vi "CreateNotifiers.vi"(8 "error in":errorcluster) -> (0 "error out":errorcluster, 3 "Notifiers":T1)   [LabVIEW 2015]
uses:
  Notifiers.ctl
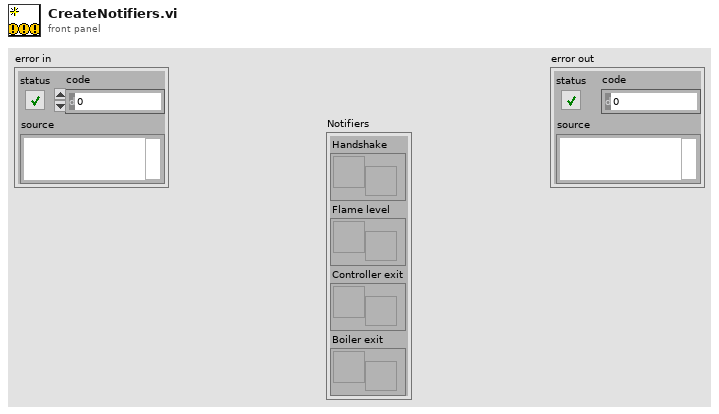
[diagram p1: front panel]
types:
  T1 = typedef "Notifiers.ctl" = cluster{"Handshake":refnum<notifier>, "Flame level":refnum<notifier>, "Controller exit":refnum<notifier>, "Boiler exit":refnum<notifier>}
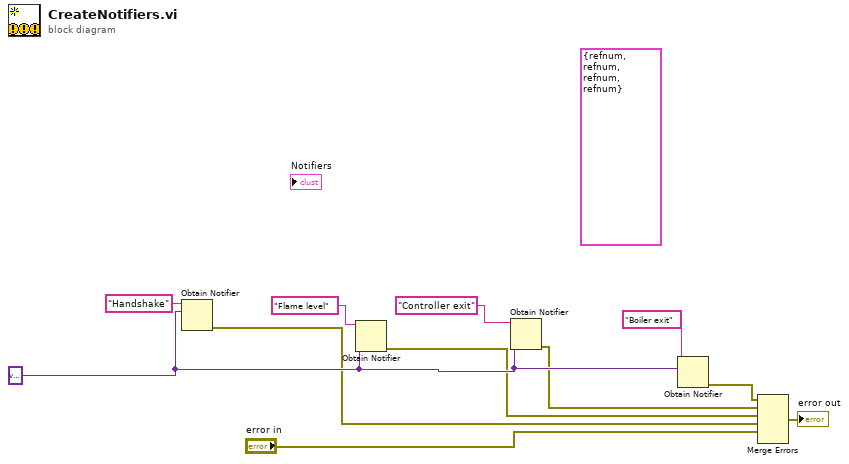
[diagram p0: block diagram]
diagram:
  (unwired) T1 {"Handshake"=refnum, "Flame level"=refnum, "Controller exit"=refnum, "Boiler exit"=refnum}
  w7 = variant
  n1 = Obtain Notifier(name (unnamed)="Handshake", notification data type=w7) -> (error out=w3:errorcluster)  [unwired: 2 in, 2 out]
  n2 = Obtain Notifier(name (unnamed)="Flame level", notification data type=w7) -> (error out=w4:errorcluster)  [unwired: 2 in, 2 out]
  n3 = Obtain Notifier(name (unnamed)="Controller exit", notification data type=w7) -> (error out=w5:errorcluster)  [unwired: 2 in, 2 out]
  n4 = Obtain Notifier(name (unnamed)="Boiler exit", notification data type=w7) -> (error out=w6:errorcluster)  [unwired: 2 in, 2 out]
  n5 = Merge Errors(w6, w5, w4, w3, "error in") -> (→"error out":errorcluster)  [unwired: 1 in]
